vi "Get Templates Folder Location.vi"() -> (0 "Templates Folder Location":path)   [LabVIEW 2021]
doc: "Returns the folder location where template VIs and/or CTLs are expected to be found."
uses:
  <vilib>/Utility/sysdir.llb/System Directory Type.ctl
panel:
  # "Development\ncontrols/indicators useful for development and testing, but which are not outputs of the VI"
  # "Input\nInputs to the VI"
  # "Output\nOutputs of the VI"
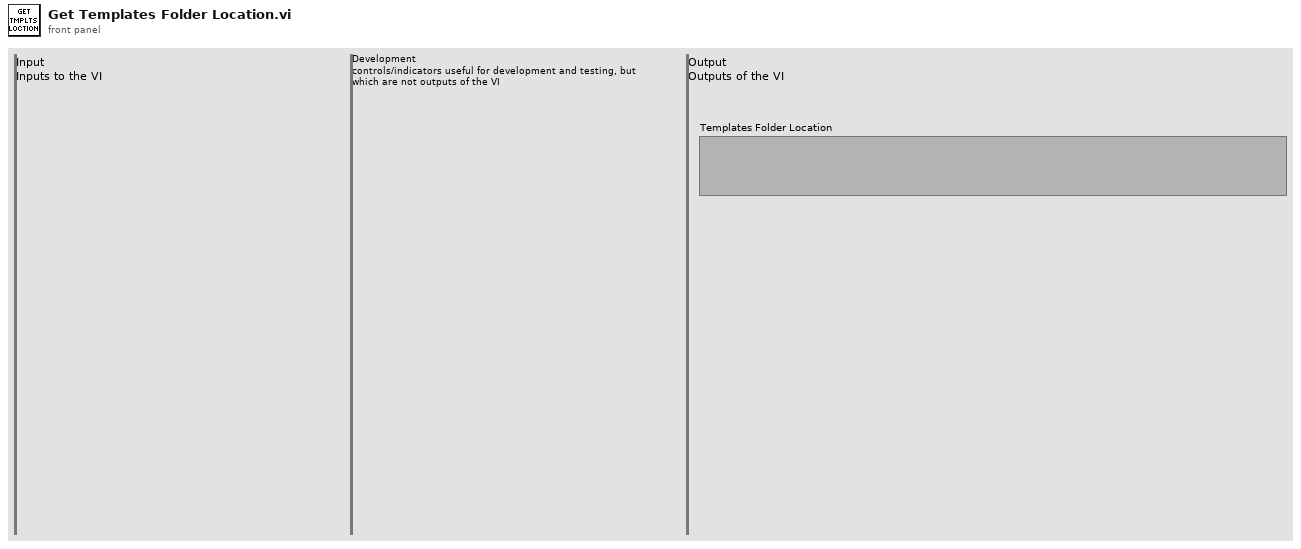
[diagram p1: front panel]
types:
  T1 = typedef "System Directory Type.ctl" = i32
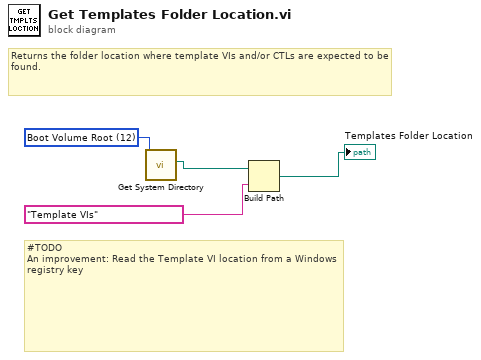
[diagram p0: block diagram]
diagram:
  w4 = T1 12 items=["User Home"=0, "User Desktop"=1, "User Documents"=2, "User Application Data"=3, "User Preferences"=4, "User Temporary"=5, "Public Documents"=6, "Public Application Data"=7, "Public Preferences"=8, "Public Cache"=13, "System Core Libraries"=9, "System Installed Libraries"=10, "Application Files"=11, "Boot Volume Root"=12] ("system directory type")
  # "#TODO\nAn improvement: Read the Template VI location from a Windows registry key"
  # "Returns the folder location where template VIs and/or CTLs are expected to be found."
  n1 = call <vilib>:"Get System Directory.vi"("system directory type"=w4) -> ("system directory"=w3:path)  [unwired: 10 in]
  n2 = Build Path(base path=w3, name or relative path="Template VIs") -> (appended path=→"Templates Folder Location":path)
